vi "labviewParse.vi"() -> ()   [LabVIEW 2021]
panel:
  out "error out":errorcluster
  in  "error in (no error)":errorcluster
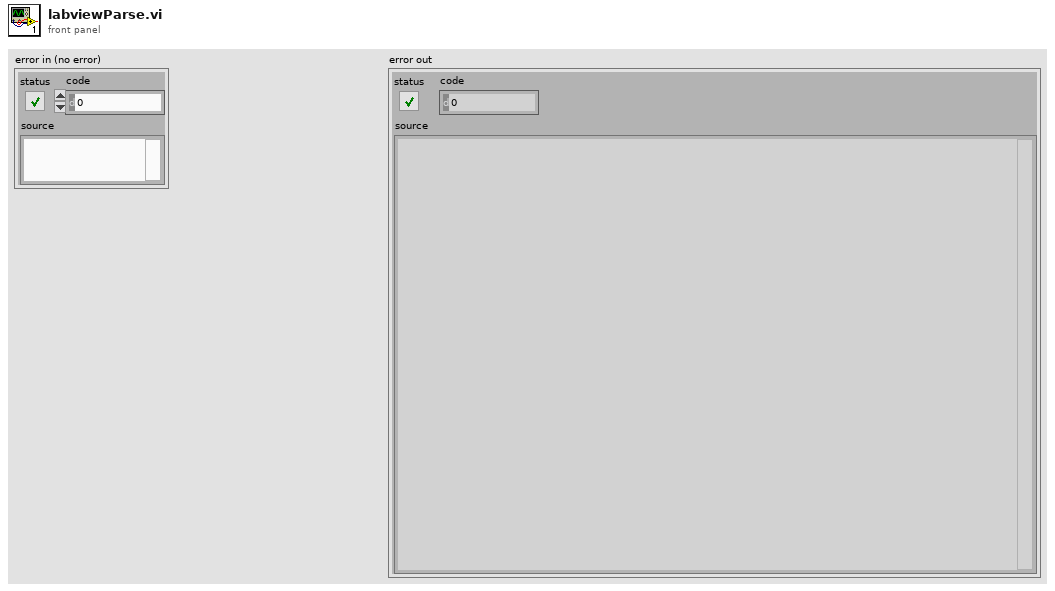
[diagram p1: front panel]
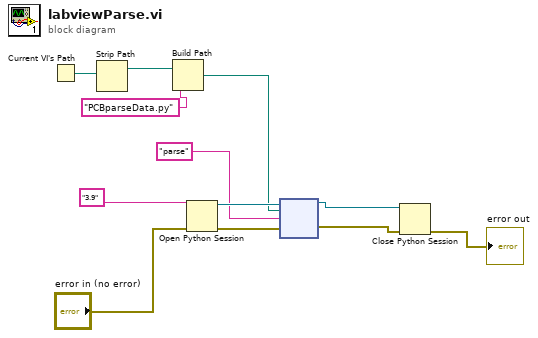
[diagram p0: block diagram]
diagram:
  n1 = Current VI's Path() -> (path=w3:path)
  n2 = Strip Path(path=w3) -> (stripped path=w9:path)  [unwired: 1 out]
  n3 = Build Path(base path=w9, name or relative path="PCBparseData.py") -> (appended path=w7:path)
  n4 = Open Python Session(python version="3.9", 3:"error in (no error)") -> (session out=w11:refnum<k35>, error out=w10:errorcluster)  [unwired: 1 in]
  n5 = node(w11, w7, "parse" ("function name"), w10) -> (w6:refnum<k35>, w5:errorcluster)  [unwired: 2 in, 2 out]
  n6 = Close Python Session(session in=w6, error in=w5) -> (11:→"error out":errorcluster)
